vi "Configure Output Mode Core.vi"(8 "error in (no error)":errorcluster, 9 "output mode (Standard Function)":i32(ring) items=["Standard Function", "Arbitrary Waveform", "Arbitrary Sequence"], 11 "CS++Fgen in":refnum<class "CS++Fgen.lvclass">) -> (0 "error out":errorcluster, 3 "CS++Fgen out":refnum<class "CS++Fgen.lvclass">)   [LabVIEW 2013, in "CS++Fgen.lvlib" / "CS++Fgen.lvclass"]
doc: "This VI configures the output mode of the function generator. The output mode determines the kind of waveform the function generator produces. For example, you can select to output a standard waveform, an arbitrary waveform, or a sequence of arbitrary waveforms."
uses:
  CS++Fgen.lvclass
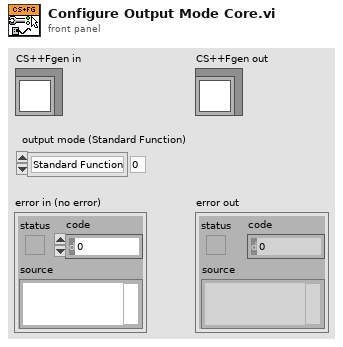
[diagram p1: front panel]
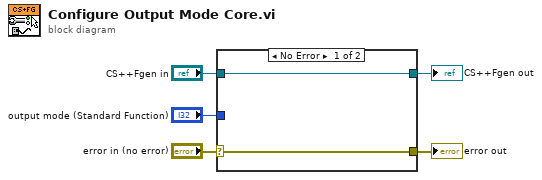
[diagram p0: block diagram]
diagram:
  n1 = case shown="No Error" "error in (no error)" {
    selector: "error in (no error)" -> [w6 w9]
    tunnel: [w6 w9] -> w4
    tunnel: [w7 w8] -> w2
    tunnel: "CS++Fgen in" -> [w7 w8]
    tunnel: "output mode (Standard Function)" -> [_ _]
    frame No Error {
    }
    frame Error {
    }
  }
  "error out" <- w4
  "CS++Fgen out" <- w2
